vi "Do Request.vi"(7 "Processing In":refnum<class "Processing.lvclass">, 11 "DebugHTTPController in":refnum<class "DebugHTTPController.lvclass">) -> (0 "error out":errorcluster, 5 "Processing":refnum<class "Processing.lvclass">)   [LabVIEW 2020, in "Volatus.lvlib" / "DebugHTTPController.lvclass"]
doc: "A controller's main job is to respond to a request by generating a response. The response value must be specified by calling Set Response.vi on the Processing class that's passed through the VI otherwise an error will be generated.\n\nThere are several helpers available for common response types:\nGenerating HTML content programmatically - Create Basic Response.vi\nStreaming a file from disk - Create File Response.vi\nRedirecting the user to another URL - Create Redirect Response.vi\n\nFile responses are streamed in chunks and do not load the entire file into memory at once to send in the response which allows serving large files more efficiently."
uses:
  DebugHTTPController.lvclass
  lv-http-server/HTTP Server/Processing/Processing.lvclass
  DebugHTTPController.lvclass/DebugHTTPController.ctl
  lv-http-server/HTTP Server/Processing/Processing.lvclass/Processing.ctl
  lv-http-util/HTTP Utils/Request/Get Target URI.vi
  lv-stream/stream/URI/Get Path.vi
  MessageQ/MessageQ.lvclass
  PathValue/PathValue.lvclass
  lv-http-util/HTTP Utils/File Response/File Response.lvclass
  lv-http-util/HTTP Utils/Response/Response.lvclass
  C:/dev/lv20CE/relink/lv-promises/Promises/Value/Value.lvclass
  C:/dev/lv20CE/relink/lv-volatus/Volatus/PathValue/PathValue.lvclass
  C:/dev/lv20CE/relink/lv-http-util/HTTP Utils/Streamable Response/Streamable Response.lvclass
  C:/dev/lv20CE/relink/lv-http-util/HTTP Utils/Response/Response.lvclass
  C:/dev/lv20CE/relink/lv-http-util/HTTP Utils/File Response/File Response.lvclass
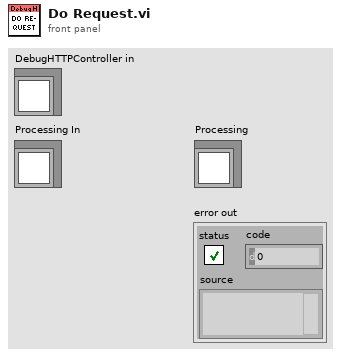
[diagram p1: front panel]
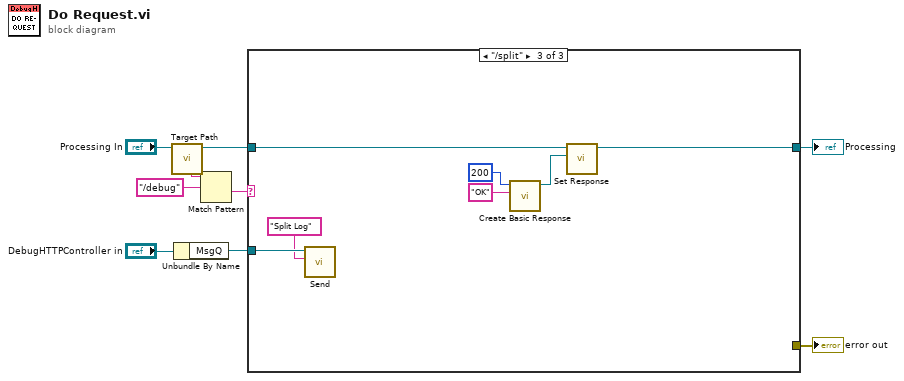
[diagram p0: block diagram]
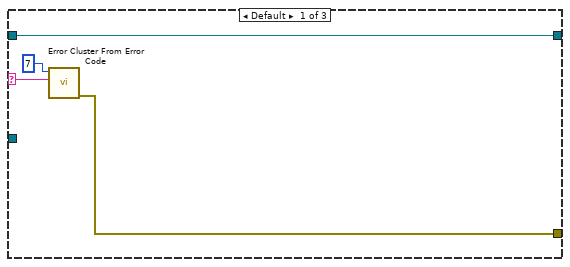
[diagram p2: hidden frame]
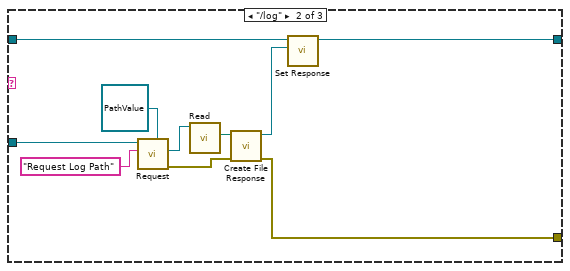
[diagram p3: hidden frame]
diagram:
  n1 = call "Target Path.vi"("Processing in"="Processing In") -> ("Processing out"=w5:refnum<class "Processing.lvclass">, "Target Path"=w9:string)  [unwired: 9 in]
  n2 = Unbundle By Name("DebugHTTPController in") -> ("MsgQ"=w1:refnum<class "MessageQ.lvclass">)
  n3 = Match Pattern(string=w9, regular expression="/debug") -> (after substring=w6:string)  [unwired: 1 in, 3 out]
  n4 = case shown="\"/split\"" w6 {
    selector: w6 -> [w13 _ _]
    tunnel: w5 -> [w11 w23 w30]
    tunnel: [w11 w15 w25] -> w4
    tunnel: [w10 w16 _] -> w3
    tunnel: w1 -> [_ w22 w29]
    frame Default {
      n5 = call <vilib>:"Error Cluster From Error Code.vi"("error message (\"\")"=w13, "error code (0)"=7) -> ("error out"=w10:errorcluster)  [unwired: 7 in]
    }
    frame "/log" {
      n6 = call "Request.vi"("Response Value Type"=refnum<class "PathValue.lvclass"> refnum ("Volatus:PathValue.lvclass"), "ID"="Request Log Path", "MessageQ in"=w22) -> ("error out"=w17:errorcluster, "Response"=w19:refnum<class "PathValue.lvclass">)  [unwired: 6 in, 1 out]
      n7 = call "Read.vi"("PathValue in"=w19) -> ("Path"=w18:path)  [unwired: 10 in]
      n8 = call "Create File Response.vi"("error in (no error)"=w17, "Path"=w18) -> ("error out"=w16:errorcluster, "File Response out"=w14:refnum<class "File Response.lvclass">)  [unwired: 8 in]
      n9 = call "Set Response.vi"("Response"=w14, "Processing in"=w23) -> ("Processing out"=w15:refnum<class "Processing.lvclass">)  [unwired: 9 in]
    }
    frame "/split" {
      n10 = call "Send.vi"("ID"="Split Log", "MessageQ in"=w29) -> ()  [unwired: 8 in, 2 out]
      n11 = call "Create Basic Response.vi"("Payload"="OK", "Status Code"=u16 200) -> ("Response out"=w24:refnum<class "Response.lvclass">)  [unwired: 8 in, 1 out]
      n12 = call "Set Response.vi"("Response"=w24, "Processing in"=w30) -> ("Processing out"=w25:refnum<class "Processing.lvclass">)  [unwired: 9 in]
    }
  }
  "error out" <- w3
  "Processing" <- w4
